vi "Pickup State Machine.vi"   [LabVIEW 2013]
uses:
  typedefs/fg_typedef.ctl
  typedefs/subStates.ctl
panel:
  # "A State Machine to Handle Pickup for Passing"
types:
  T1 = typedef "subStates.ctl" = enum16{"null", "wait", "driver control", "auto", "manual override", "hold position", "rotate", "pickup", "pass", "load", "goto shoot", "shoot high goal", "shoot low goal", "cancel arm", "cancel shooter", "end"}
  T2 = typedef "fg_typedef.ctl" = enum16{"Get", "Set"}
  T3 = enum16{"Shooter Solenoid", "Latch Solenoid", "Right Up Sensor", "Right Down Sensor", "Hold Sensor"}
  T4 = typedef "WPI_DigitalInputDevRef.ctl" = cluster{"DevStatus":errorcluster, "DIO Channel":T5, "Digital Module":T6}
  T5 = typedef "FPGA_DIOChannel.ctl" = enum8{"DIO 1", "DIO 2", "DIO 3", "DIO 4", "DIO 5", "DIO 6", "DIO 7", "DIO 8", "DIO 9", "DIO 10", "DIO 11", "DIO 12", "DIO 13", "DIO 14", "Invalid"}
  T6 = typedef "FPGA_TypedefDigitalModule.ctl" = enum16{"Digital Module 1", "Digital Module 2"}
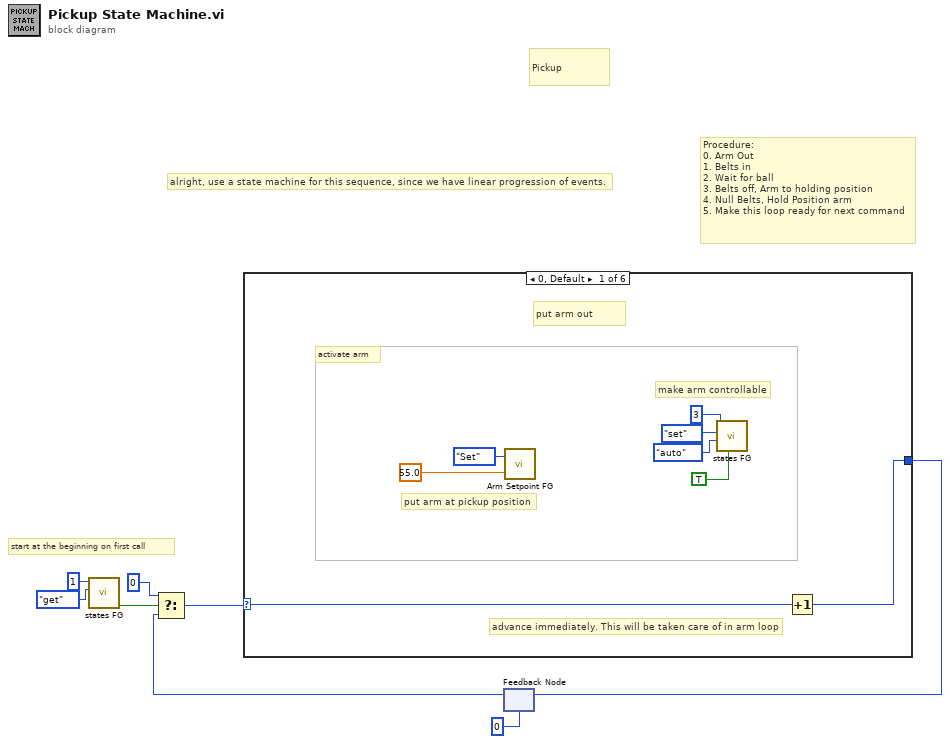
[diagram p0: block diagram]
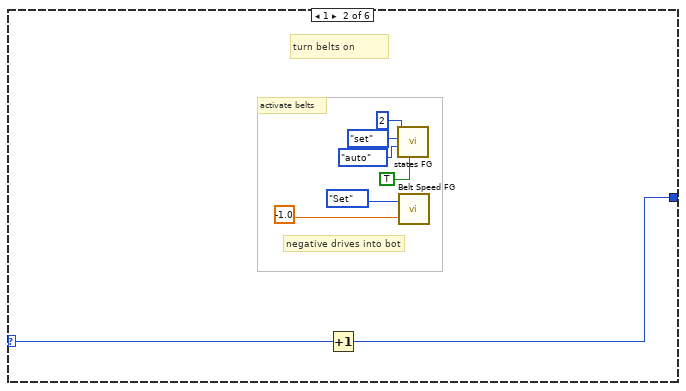
[diagram p2: hidden frame]
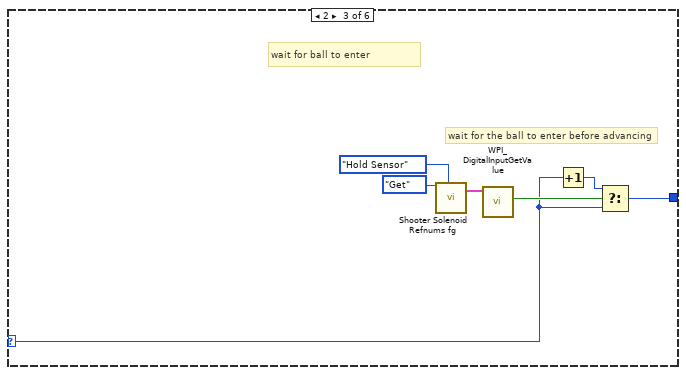
[diagram p3: hidden frame]
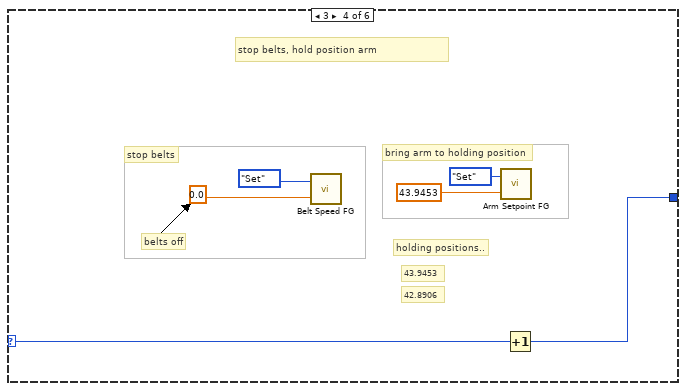
[diagram p4: hidden frame]
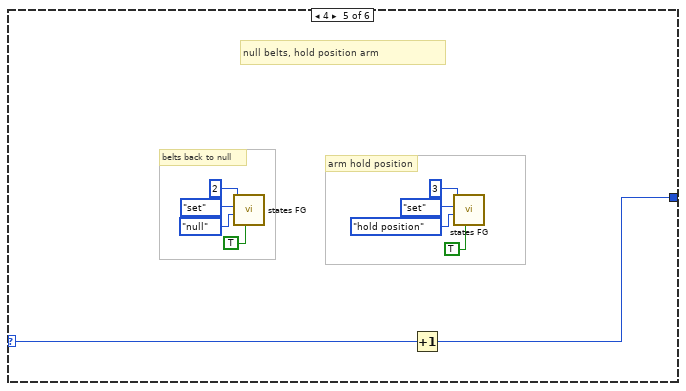
[diagram p5: hidden frame]
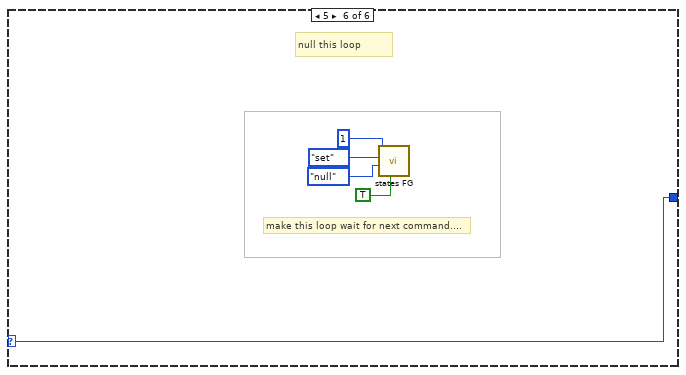
[diagram p6: hidden frame]
diagram:
  # "start at the beginning on first call"
  # "Pickup"
  # "Procedure: \n0. Arm Out\n1. Belts in\n2. Wait for ball\n3. Belts off, Arm to holding position\n4. Null Belts, Hold Position arm\n5. Make this loop ready for next command"
  # "alright, use a state machine for this sequence, since we have linear progression of events."
  n1 = call "states FG.vi"("menu (get)"=enum16{"set", "get"}."get", "Loop ID"=1) -> ("first call?"=w1:bool)  [unwired: 6 in, 3 out]
  n2 = feedback #1(u8 0) -> (w2:u8)
  n3 = Select(t=u8 0, s=w1, f=w2) -> (s? t:f=w4:u8)
  n4 = case shown="0, Default" w4 {
    selector: w4 -> [w11 w19 w29 w33 w41 w49]
    tunnel: [w10 w18 w28 w32 w40 w49] -> w7
    frame 0, Default {
      # "put arm at pickup position"
      # "activate arm"
      # "make arm controllable"
      # "advance immediately. This will be taken care of in arm loop"
      # "put arm out"
      n5 = call "Arm Setpoint FG.vi"("Setpoint In"=55.0, "Menu"=fg_typedef."Set") -> ()  [unwired: 1 out]
      n6 = call "states FG.vi"("exit in"=TRUE, "subState in"=subStates."auto", "menu (get)"=enum16{"set", "get"}."set", "Loop ID"=3) -> ()  [unwired: 4 in, 4 out]
      n7 = Increment(x=w11) -> (x+1=w10:u8)
    }
    frame 1 {
      # "activate belts"
      # "negative drives into bot"
      # "turn belts on"
      n8 = Increment(x=w19) -> (x+1=w18:u8)
      n9 = call "states FG.vi"("exit in"=TRUE, "subState in"=subStates."auto", "menu (get)"=enum16{"set", "get"}."set", "Loop ID"=2) -> ()  [unwired: 4 in, 4 out]
      n10 = call "Belt Speed FG.vi"("Speed In"=-1.0 ("Setpoint In"), "Menu"=fg_typedef."Set") -> ()  [unwired: 1 out]
    }
    frame 2 {
      # "wait for ball to enter"
      # "wait for the ball to enter before advancing"
      n11 = call "Shooter Solenoid Refnums fg.vi"("Menu"=fg_typedef."Get", "DevRef to Get"=T3."Hold Sensor") -> ("Selected Sensor"=w26:T4)  [unwired: 16 in, 1 out]
      n12 = call <vilib>:"WPI_DigitalInputGetValue.vi"("DigitalInputDevRef"=w26) -> ("Value"=w30:bool)  [unwired: 8 in, 2 out]
      n13 = Increment(x=w29) -> (x+1=w31:u8)
      n14 = Select(t=w31, s=w30, f=w29) -> (s? t:f=w28:u8)
    }
    frame 3 {
      # "stop belts, hold position arm"
      # "42.8906"
      # "holding positions.."
      # "43.9453"
      # "stop belts"
      # "bring arm to holding position"
      # "belts off"
      n15 = call "Belt Speed FG.vi"("Speed In"=0.0 ("Setpoint In"), "Menu"=fg_typedef."Set") -> ()  [unwired: 1 out]
      n16 = call "Arm Setpoint FG.vi"("Setpoint In"=43.9453, "Menu"=fg_typedef."Set") -> ()  [unwired: 1 out]
      n17 = Increment(x=w33) -> (x+1=w32:u8)
    }
    frame 4 {
      # "arm hold position"
      # "belts back to null"
      # "null belts, hold position arm"
      n18 = call "states FG.vi"("exit in"=TRUE, "subState in"=subStates."null", "menu (get)"=enum16{"set", "get"}."set", "Loop ID"=2) -> ()  [unwired: 4 in, 4 out]
      n19 = Increment(x=w41) -> (x+1=w40:u8)
      n20 = call "states FG.vi"("exit in"=TRUE, "subState in"=subStates."hold position", "menu (get)"=enum16{"set", "get"}."set", "Loop ID"=3) -> ()  [unwired: 4 in, 4 out]
    }
    frame 5 {
      # "null this loop"
      # "make this loop wait for next command...."
      n21 = call "states FG.vi"("exit in"=TRUE, "subState in"=subStates."null", "menu (get)"=enum16{"set", "get"}."set", "Loop ID"=1) -> ()  [unwired: 4 in, 4 out]
    }
  }
  n22 = feedback-in #1(w7) -> ()
